vi "电阻数组均值.vi"(1 "电阻数组":dbl[][](array[numeric])) -> (0 "均值":string[](array[string]))   [LabVIEW 2015]
uses:
  <vilib>/Analysis/baseanly.llb/Mean (DBL).vi
  <vilib>/Analysis/NI_AALBase.lvlib
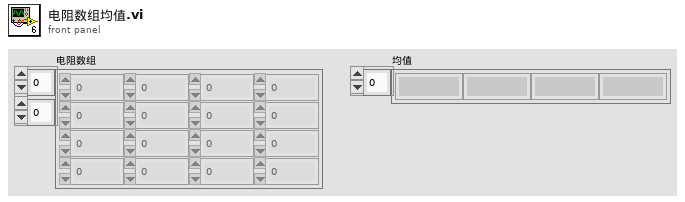
[diagram p1: front panel]
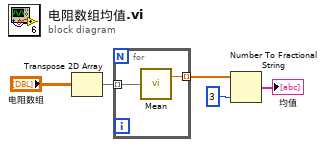
[diagram p0: block diagram]
diagram:
  n1 = Transpose 2D Array(2D array="电阻数组") -> (transposed array=w4:dbl[][])
  n2 = for {
    tunnel: w4 -> [w7] mode=indexing
    tunnel: [w6] -> w3 mode=indexing
    n3 = call-poly <vilib>:"Mean.vi"("X"=w7) -> ("mean"=w6:dbl)  [unwired: 1 out]
  }
  n4 = Number To Fractional String(number=w3, precision (6)=i16 3 ("精度(6)")) -> (F-format string=→"均值":string[])  [unwired: 2 in]
